vi "Initialize Actor.vi"(7 "Host Name":string, 8 "error in (no error)":errorcluster, 9 "Actor Name":string, 10 "Message Broker Interface":refnum<class "Message Broker Interface.lvclass">, 11 "Car Position Simulator in":refnum<class "Car Position Simulator.lvclass">) -> (0 "error out":errorcluster, 3 "Car Position Simulator out":refnum<class "Car Position Simulator.lvclass">)   [LabVIEW 2016, in "CLD Exam - Car Wash.lvlib" / "Car Position Simulator.lvclass"]
doc: "--\nCopyright © 2017 Composed SystemsI All rights reserved.\n\nAuthor: Jon McBee <jon.mcbee@composed.io>\n\nThis library is provided \"AS IS\" ,WITHOUT WARRANTIES OR\nCONDITIONS OF ANY KIND, either express or implied.\n\nComposed Systems -- composed.io\n\nStream 0.0.1.1\nJon McBee - Composed Systems\nCopyright (c) 2017, Composed Systems"
uses:
  Car Position Simulator.lvclass
  Mediator/Classes/Message Broker Interface/Message Broker Interface.lvclass
  Car Position Simulator.lvclass/Car Position Simulator.ctl
  Mediator/Classes/Message Transport Event/Message Transport Event.lvclass
  D:/Repos/Stream/software/Mediator/Classes/Message Transport Interface/Message Transport Interface.lvclass
  Mediator/Classes/Mediated Synchronous Actor/Mediated Synchronous Actor.lvclass
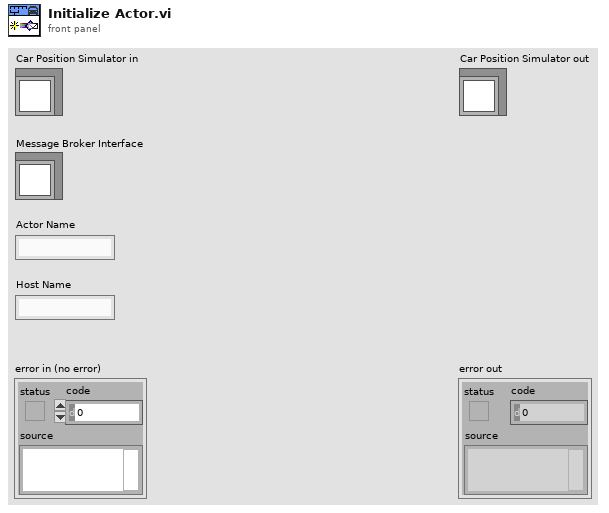
[diagram p1: front panel]
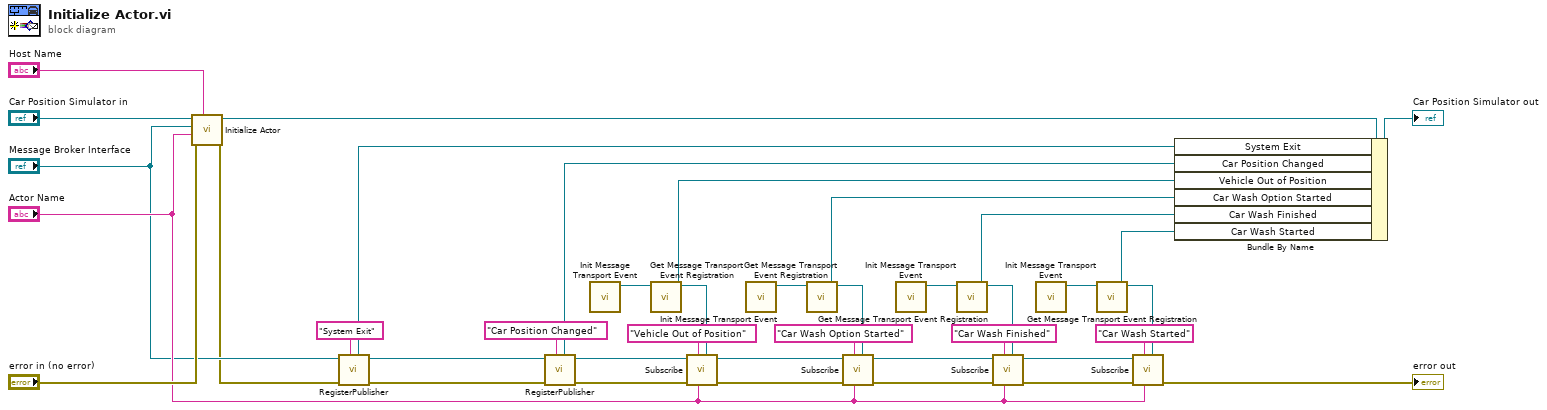
[diagram p0: block diagram]
diagram:
  n1 = call-parent "Initialize Actor.vi"("Host Name"="Host Name", "error in (no error)"="error in (no error)", "Actor Name"="Actor Name", "Message Broker Interface"="Message Broker Interface", "Mediated Synchronous Actor in"="Car Position Simulator in") -> ("error out"=w3:errorcluster, "Mediated Synchronous Actor out"=w36:refnum<class "Car Position Simulator.lvclass">)  [unwired: 5 in]
  n2 = call-dynamic "RegisterPublisher.vi"("Topic Name"="System Exit", "error in (no error)"=w3, "Message Broker Interface in"="Message Broker Interface") -> ("error out"=w2:errorcluster, "Message Broker Interface out"=w4:refnum<class "Message Broker Interface.lvclass">, "Transport"=w1:refnum<class "Message Transport Queue.lvclass">)  [unwired: 4 in, 2 out]
  n3 = call-dynamic "RegisterPublisher.vi"("Topic Name"="Car Position Changed", "error in (no error)"=w2, "Message Broker Interface in"=w4) -> ("error out"=w33:errorcluster, "Message Broker Interface out"=w32:refnum<class "Message Broker Interface.lvclass">, "Transport"=w28:refnum<class "Message Transport Queue.lvclass">)  [unwired: 4 in, 2 out]
  n4 = call "Init Message Transport Event.vi"() -> ("Message Transport Event out"=w31:refnum<class "Message Transport Event.lvclass">)  [unwired: 10 in, 1 out]
  n5 = call "Get Message Transport Event Registration.vi"("Message Transport Event in"=w31) -> ("Event Registration Refnum"=w27:refnum<event-registration>, "Message Transport Event out"=w29:refnum<class "Message Transport Event.lvclass">)  [unwired: 7 in, 2 out]
  n6 = call-dynamic "Subscribe.vi"("Message Transport Interface"=w29, "Subscriber Name"="Actor Name", "Topic Name"="Vehicle Out of Position", "error in (no error)"=w33, "Message Broker Interface in"=w32) -> ("error out"=w22:errorcluster, "Message Broker Interface out"=w23:refnum<class "Message Broker Interface.lvclass">)  [unwired: 4 in, 1 out]
  n7 = call "Init Message Transport Event.vi"() -> ("Message Transport Event out"=w24:refnum<class "Message Transport Event.lvclass">)  [unwired: 10 in, 1 out]
  n8 = call "Get Message Transport Event Registration.vi"("Message Transport Event in"=w24) -> ("Event Registration Refnum"=w21:refnum<event-registration>, "Message Transport Event out"=w26:refnum<class "Message Transport Event.lvclass">)  [unwired: 7 in, 2 out]
  n9 = call-dynamic "Subscribe.vi"("Message Transport Interface"=w26, "Subscriber Name"="Actor Name", "Topic Name"="Car Wash Option Started", "error in (no error)"=w22, "Message Broker Interface in"=w23) -> ("error out"=w18:errorcluster, "Message Broker Interface out"=w17:refnum<class "Message Broker Interface.lvclass">)  [unwired: 4 in, 1 out]
  n10 = call "Init Message Transport Event.vi"() -> ("Message Transport Event out"=w20:refnum<class "Message Transport Event.lvclass">)  [unwired: 10 in, 1 out]
  n11 = call "Get Message Transport Event Registration.vi"("Message Transport Event in"=w20) -> ("Event Registration Refnum"=w15:refnum<event-registration>, "Message Transport Event out"=w19:refnum<class "Message Transport Event.lvclass">)  [unwired: 7 in, 2 out]
  n12 = call-dynamic "Subscribe.vi"("Message Transport Interface"=w19, "Subscriber Name"="Actor Name", "Topic Name"="Car Wash Finished", "error in (no error)"=w18, "Message Broker Interface in"=w17) -> ("error out"=w11:errorcluster, "Message Broker Interface out"=w8:refnum<class "Message Broker Interface.lvclass">)  [unwired: 4 in, 1 out]
  n13 = call "Init Message Transport Event.vi"() -> ("Message Transport Event out"=w12:refnum<class "Message Transport Event.lvclass">)  [unwired: 10 in, 1 out]
  n14 = call "Get Message Transport Event Registration.vi"("Message Transport Event in"=w12) -> ("Event Registration Refnum"=w7:refnum<event-registration>, "Message Transport Event out"=w13:refnum<class "Message Transport Event.lvclass">)  [unwired: 7 in, 2 out]
  n15 = call-dynamic "Subscribe.vi"("Message Transport Interface"=w13, "Subscriber Name"="Actor Name", "Topic Name"="Car Wash Started", "error in (no error)"=w11, "Message Broker Interface in"=w8) -> ("error out"=→"error out":errorcluster)  [unwired: 4 in, 2 out]
  n16 = Bundle By Name(cluster=w36, "System Exit"=w1, "Car Position Changed"=w28, "Vehicle Out of Position"=w27, "Car Wash Option Started"=w21, "Car Wash Finished"=w15, "Car Wash Started"=w7) -> (→"Car Position Simulator out":refnum<class "Car Position Simulator.lvclass">)
